vi "Read Multipage ImageJ TIFF Frame.vi"(0 "TIF Ref":refnum<file>, 7 "Image Info":T1, 11 "Error":errorcluster, 13 "Frame":u32) -> (2 "U8 Image":u8[][](array[numeric]), 4 "TIF Ref (Dup)":refnum<file>, 8 "U16 Image":u16[][](array[numeric]), 15 "Error":errorcluster)   [LabVIEW 2020]
doc: "Reads a single frame from a multipage (stack) ImageJ TIF image. The file must already be open and header info provided by \"Read Multipage ImageJ TIFF Header.vi.\" The first frame is the 0th frame. Be sure to close the file reference when done."
uses:
  ImageJ TIF Type Defs/TIF Read Image Information.ctl
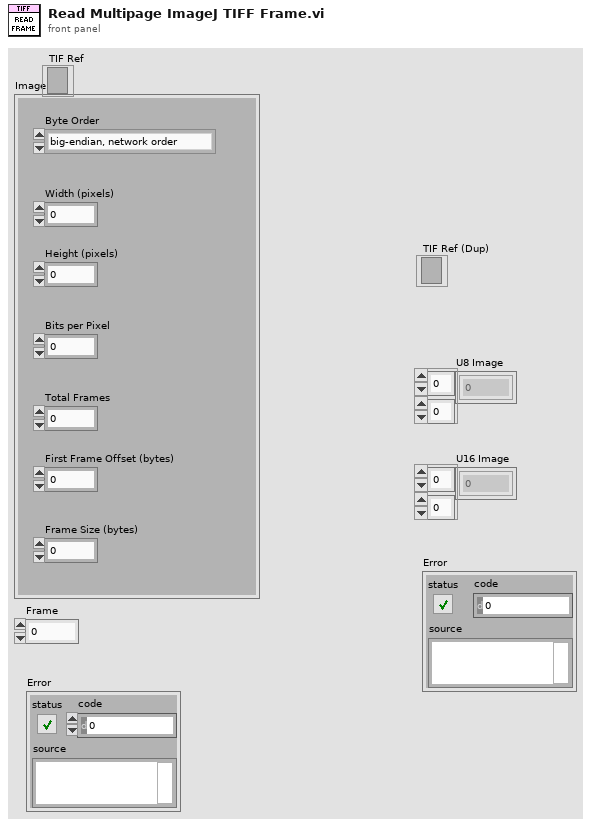
[diagram p1: front panel]
types:
  T1 = typedef "TIF Read Image Information.ctl" = cluster{"Byte Order":enum16{"big-endian, network order", "native, host order", "little-endian"}, "Width (pixels)":i32, "Height (pixels)":i32, "Bits per Pixel":u8, "Total Frames":u32, "First Frame Offset (bytes)":u32, "Frame Size (bytes)":u32}
  T2 = enum16{"big-endian, network order", "native, host order", "little-endian"}
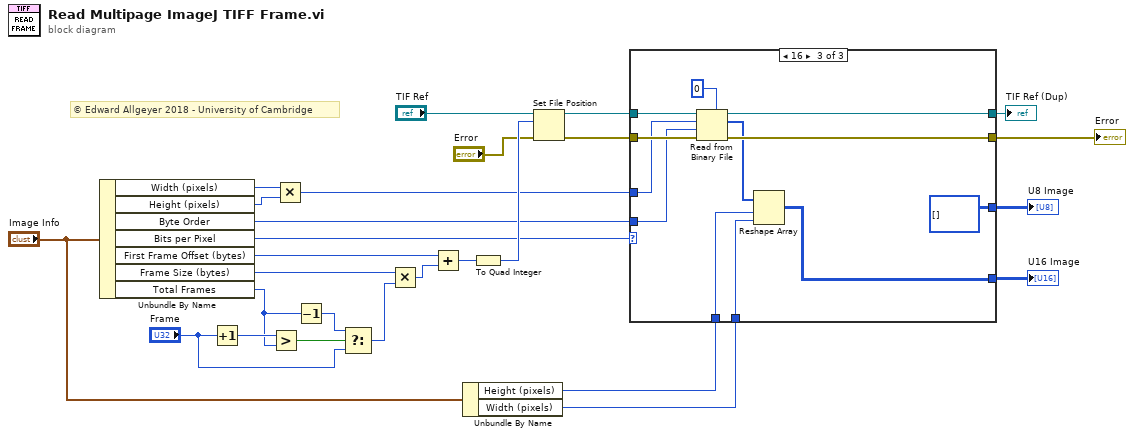
[diagram p0: block diagram]
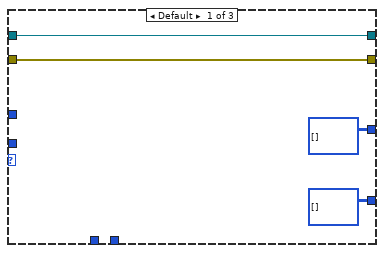
[diagram p2: hidden frame]
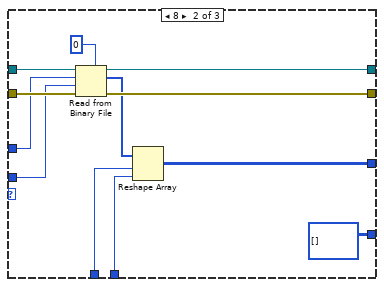
[diagram p3: hidden frame]
diagram:
  # "© Edward Allgeyer 2018 - University of Cambridge"
  n1 = Unbundle By Name("Image Info") -> ("Width (pixels)"=w10:i32, "Height (pixels)"=w9:i32, "Byte Order"=w8:T2, "Bits per Pixel"=w14:u8, "First Frame Offset (bytes)"=w25:u32, "Frame Size (bytes)"=w24:u32, "Total Frames"=w18:u32)
  n2 = Increment(x="Frame") -> (x+1=w19:u32)
  n3 = Greater?(x=w19, y=w18) -> (0:w20:bool)
  n4 = Multiply(x=w10, y=w9) -> (x*y=w11:i32)
  n5 = Decrement(x=w18) -> (x-1=w17:u32)
  n6 = Select(t=w17, s=w20, f="Frame") -> (s? t:f=w15:u32)
  n7 = Multiply(x=w24, y=w15) -> (x*y=w23:u32)
  n8 = Add(x=w25, y=w23) -> (x+y=w22:u32)
  n9 = Unbundle By Name("Image Info") -> ("Height (pixels)"=w6:i32, "Width (pixels)"=w5:i32)
  n10 = To Quad Integer(1:w22) -> (0:w21:i64)
  n11 = Set File Position(offset (in bytes) (0)=w21, refnum="TIF Ref", error in="Error") -> (refnum out=w26:refnum<file>, error out=w13:errorcluster)  [unwired: 1 in]
  n12 = case shown="16" w14 {
    tunnel: w26 -> [w31 w43 w55]
    tunnel: w13 -> [w30 w41 w53]
    tunnel: w11 -> [_ w40 w52]
    tunnel: w8 -> [_ w39 w51]
    tunnel: [w31 w38 w50] -> w2
    tunnel: [w30 w37 w49] -> w1
    tunnel: w6 -> [_ w35 w47]
    tunnel: w5 -> [_ w34 w46]
    tunnel: [u8[][] [] w33 u8[][] []] -> w4
    tunnel: [u16[][] [] u16[][] [] w45] -> w3
    frame Default {
    }
    frame 8 {
      n13 = Read from Binary File(5:u8 0, 8:w41, 9:w39, 10:w40, 11:w43) -> (0:w37:errorcluster, 2:w36:u8[], 3:w38:refnum<file>)  [unwired: 1 in, 1 out]
      n14 = Reshape Array(w36, w35, w34) -> (w33:u8[][])
    }
    frame 16 {
      n15 = Read from Binary File(5:u16 0, 8:w53, 9:w51, 10:w52, 11:w55) -> (0:w49:errorcluster, 2:w48:u16[], 3:w50:refnum<file>)  [unwired: 1 in, 1 out]
      n16 = Reshape Array(w48, w47, w46) -> (w45:u16[][])
    }
  }
  "U8 Image" <- w4
  "U16 Image" <- w3
  "TIF Ref (Dup)" <- w2
  "Error" <- w1
